vi "Constant - Serial Timeout (ms).vi"() -> (3 "timeout (ms)":i32=3000)   [LabVIEW 2021]
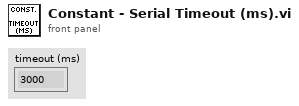
[diagram p1: front panel]
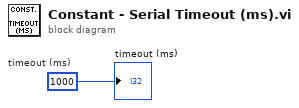
[diagram p0: block diagram]
diagram:
  w1 = 1000  # timeout (ms)
  "timeout (ms)" <- w1
